vi "Generate.vi"(0 "reference in":refnum<class "Matlab.lvclass">, 1 "Path":path, 3 "Classes":T1[](array[typedef]), 5 "error in (no error)":errorcluster) -> (14 "reference out":refnum<class "Matlab.lvclass">, 19 "error out":errorcluster)   [LabVIEW 2018, in "Matlab.lvclass"]
uses:
  Matlab.lvclass
  Executer_class/typedefs/ClassDescription.ctl
  Executer_class/typedefs/MethodDescription.ctl
  Executer_class/Executer.lvclass
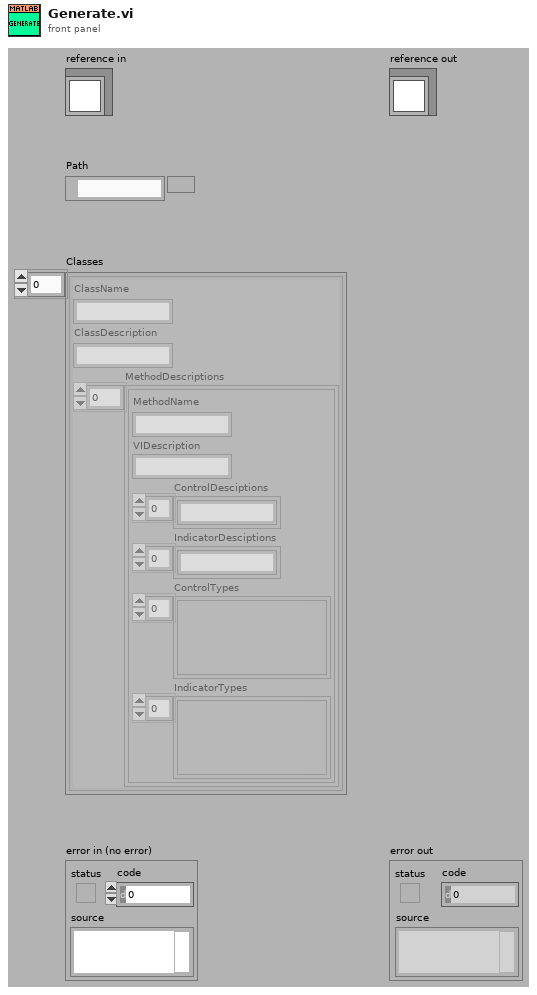
[diagram p1: front panel]
types:
  T1 = typedef "Executer.lvclass/ClassDescription.ctl" = cluster{"ClassName":string, "ClassDescription":string, "MethodDescriptions":T2[]}
  T2 = typedef "Executer.lvclass/MethodDescription.ctl" = cluster{"MethodName":string, "VIDescription":string, "ControlDesciptions":string[], "IndicatorDesciptions":string[], "ControlTypes":variant[], "IndicatorTypes":variant[]}
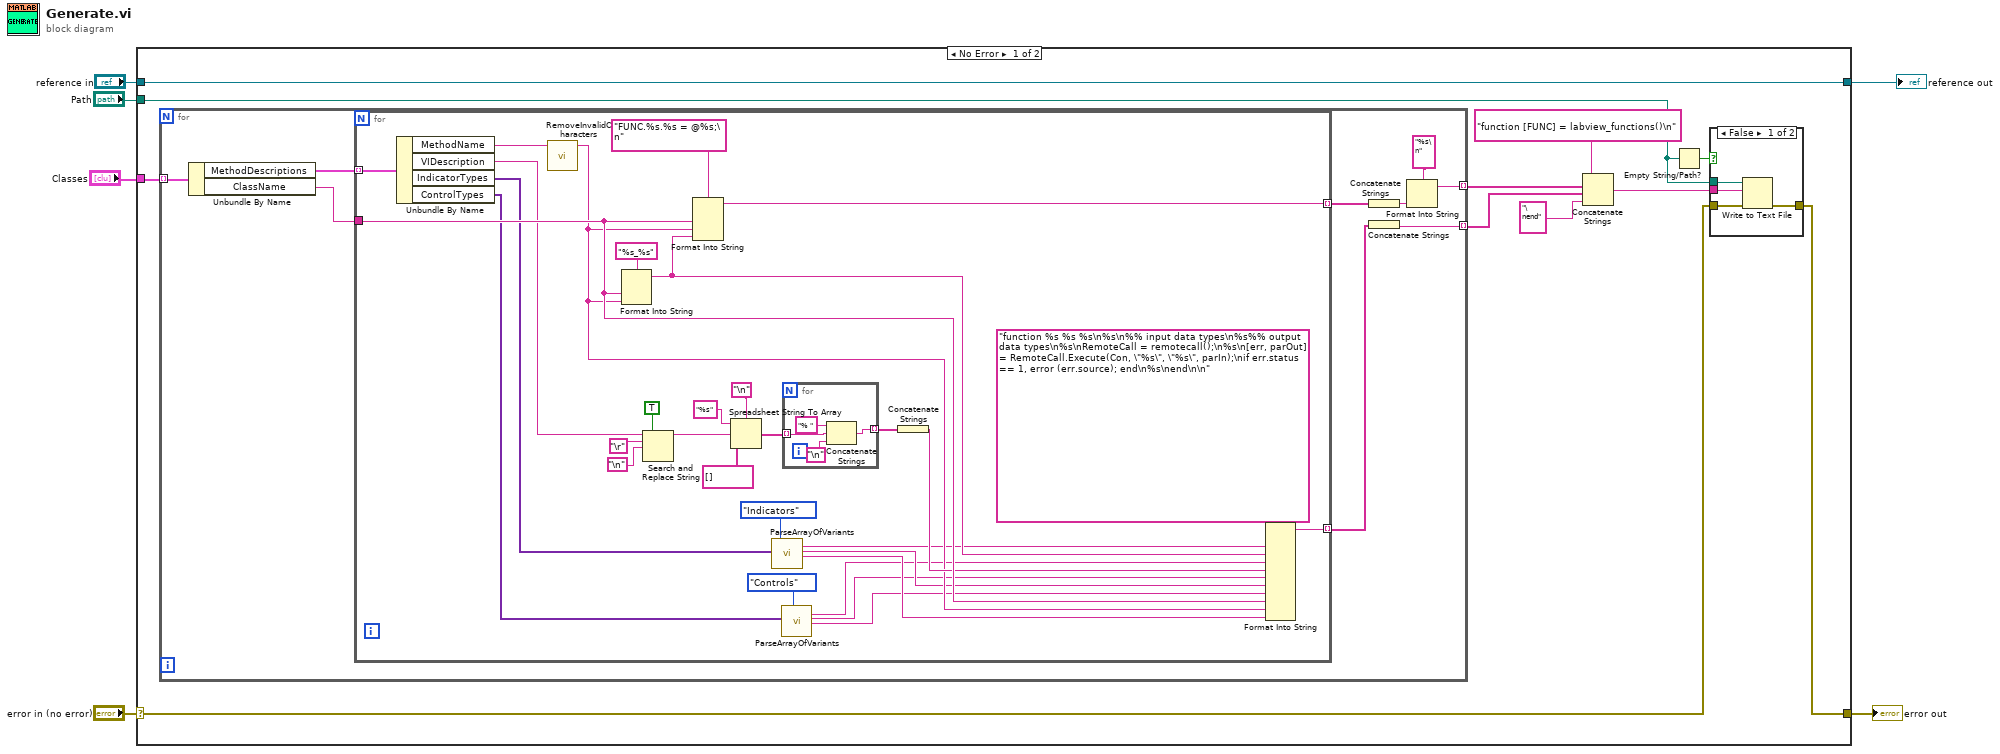
[diagram p0: block diagram]
diagram:
  n1 = case shown="No Error" "error in (no error)" {
    selector: "error in (no error)" -> [w16 w68]
    tunnel: [w7 w68] -> w5
    tunnel: [w17 w67] -> w3
    tunnel: "reference in" -> [w17 w67]
    tunnel: "Classes" -> [w9 _]
    tunnel: "Path" -> [w8 _]
    frame No Error {
      n2 = for {
        tunnel: [w22] -> w13 mode=indexing
        tunnel: [w21] -> w14 mode=indexing
        tunnel: w9 -> [w20] mode=indexing
        n3 = Unbundle By Name(w20) -> ("MethodDescriptions"=w18:T2[], "ClassName"=w19:string)
        n4 = for {
          tunnel: [w57] -> w26 mode=indexing
          tunnel: w19 -> [w55]
          tunnel: [w56] -> w25 mode=indexing
          tunnel: w18 -> [w54] mode=indexing
          n5 = Unbundle By Name(w54) -> ("MethodName"=w39:string, "VIDescription"=w37:string, "IndicatorTypes"=w36:variant[], "ControlTypes"=w35:variant[])
          n6 = call "RemoveInvalidCharacters.vi"("string in"=w39) -> ("string out"=w38:string)  [unwired: 10 in]
          n7 = Format Into String(format string="%s_%s", w55, w38) -> (resulting string=w50:string)  [unwired: 2 in, 1 out]
          n8 = Search and Replace String(replace all?=TRUE ("replace all? (F)"), input string=w37, search string="\r", replace string="\n") -> (result string=w41:string)  [unwired: 4 in, 3 out]
          n9 = Format Into String(format string="FUNC.%s.%s = @%s;\n", w55, w38, w50) -> (resulting string=w56:string)  [unwired: 2 in, 1 out]
          n10 = Spreadsheet String To Array(delimiter (Tab)="\n", format string="%s", spreadsheet string=w41, array type (2D Dbl)=string[] []) -> (array=w47:string[])
          n11 = call "ParseArrayOfVariants.vi"("Types"=w36, "Type"=enum16{"Indicators", "Controls"}."Indicators") -> ("Funcdefinition"=w32:string, "Description"=w31:string, "FuncString"=w30:string)  [unwired: 15 in]
          n12 = call "ParseArrayOfVariants.vi"("Types"=w35, "Type"=enum16{"Indicators", "Controls"}."Controls") -> ("Funcdefinition"=w29:string, "Description"=w28:string, "FuncString"=w27:string)  [unwired: 15 in]
          n13 = for {
            tunnel: w47 -> [w61] mode=indexing
            tunnel: [w59] -> w46 mode=indexing
            n14 = Concatenate Strings("% " ("string"), w61, "\n") -> (w59:string)
          }
          n15 = Concatenate Strings(w46) -> (w45:string)
          n16 = Format Into String(format string="function %s %s %s\n%s\n%% input data types\n%s%% output data types\n%s\nRemoteCall = remotecall();\n%s\n[err, parOut] = RemoteCall.Execute(Con, \"%s\", \"%s\", parIn);\nif err.status == 1, error (err.source); end\n%s\nend\n\n", w32, w50, w29, w45, w28, w31, w27, w55, w38, w30) -> (resulting string=w57:string)  [unwired: 2 in, 1 out]
        }
        n17 = Concatenate Strings(w25) -> (w23:string)
        n18 = Concatenate Strings(w26) -> (w21:string)
        n19 = Format Into String(format string="%s\n", w23) -> (resulting string=w22:string)  [unwired: 2 in, 1 out]
      }
      n20 = Concatenate Strings("function [FUNC] = labview_functions()\n" ("format string"), w13, w14, "\nend" ("format string")) -> (w15:string)
      n21 = Empty String/Path?(string/path=w8) -> (empty?=w10:bool)
      n22 = case shown="False" w10 {
        tunnel: w15 -> [w65 _]
        tunnel: w8 -> [w64 _]
        tunnel: w16 -> [w63 w66]
        tunnel: [w62 w66] -> w7
        frame False {
          n23 = Write to Text File(file (use dialog)=w64, text=w65, error in=w63) -> (error out=w62:errorcluster)  [unwired: 1 in, 2 out]
        }
        frame True {
        }
      }
    }
    frame Error {
    }
  }
  "error out" <- w5
  "reference out" <- w3
